vi "Facade.vi"(0 "Data In":T4, 2 "Display State In":T2, 3 "Container State":T3) -> (6 "Data Out":T4, 7 "Display State Out":T2, 8 "Action":T1)   [LabVIEW 2016, in "MGI Path Selector.xctl"]
doc: "Facade VI for the Path Selector XControl. This XControl allows the user to select a path using a combobox. The behavior of the XControl depends upon the LVObject used for its implementation.\n\nAuthored by Shawn Walpole\nsupport@mooregoodideas.com\nwww.mooregoodideas.com\n\nCopyright (c) 2013, Moore Good Ideas, Inc.\n\nAll rights reserved.\n\nRedistribution and use in source and binary forms, with or without modification, are permitted provided that the following conditions are met:\n\n * Redistributions of source code must retain the above copyright notice, this list of conditions and the following disclaimer.\n * Redistributions in binary form must reproduce the above copyright notice, this list of conditions and the following disclaimer in the documentation and/or other materials provided with the distribution.\n * Neither the name of Moore Good Ideas, Inc. nor the names of its contributors may be used to endorse or promote products derived from this software without specific prior written permission.\n\nTHIS SOFTWARE IS PROVIDED BY THE COPYRIGHT HOLDERS AND CONTRIBUTORS \"AS IS\" AND ANY EXPRESS OR IMPLIED WARRANTIES, INCLUDING, BUT NOT LIMITED TO, THE IMPLIED WARRANTIES OF MERCHANTABILITY AND FITNESS FOR A PARTICULAR PURPOSE ARE DISCLAIMED. IN NO EVENT SHALL THE COPYRIGHT OWNER OR CONTRIBUTORS BE LIABLE FOR ANY DIRECT, INDIRECT, INCIDENTAL, SPECIAL, EXEMPLARY, OR CONSEQUENTIAL DAMAGES (INCLUDING, BUT NOT LIMITED TO, PROCUREMENT OF SUBSTITUTE GOODS OR SERVICES; LOSS OF USE, DATA, OR PROFITS; OR BUSINESS INTERRUPTION) HOWEVER CAUSED AND ON ANY THEORY OF LIABILITY, WHETHER IN CONTRACT, STRICT LIABILITY, OR TORT (INCLUDING NEGLIGENCE OR OTHERWISE) ARISING IN ANY WAY OUT OF THE USE OF THIS SOFTWARE, EVEN IF ADVISED OF THE POSSIBILITY OF SUCH DAMAGE."
uses:
  <userlib>/_MGI/User Interface/Path Selector XControl/MGI Path Selector.xctl
  <vilib>/_xctls/Action.ctl
  <vilib>/_xctls/XControlSupport.lvlib
  <userlib>/_MGI/User Interface/Path Selector XControl/Class Hierarchy/MGI Path Selector.lvclass
  <vilib>/event_ctls.llb/lveventtype.ctl
  <userlib>/_MGI/User Interface/Path Selector XControl/Event Cluster.ctl
  <vilib>/Utility/miscctls.llb/LVPoint32TypeDef.ctl
  <vilib>/_xctls/Container State.ctl
  <userlib>/_MGI/User Interface/Path Selector XControl/Data.ctl
  <userlib>/_MGI/User Interface/Path Selector XControl/State.ctl
panel:
  in  "Silver Combo":string(combo)
  in  "Classic Combo":string(combo)
  in  "3D Combo":string(combo)
  in  "Combo Box":string(combo)
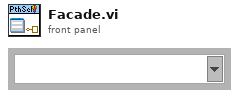
[diagram p1: front panel]
types:
  T1 = typedef "XControlSupport.lvlib/Action.ctl" = cluster{"Data Changed?":bool, "State Changed?":bool, "Action Name":string}
  T2 = typedef "MGI Path Selector.xctl/State.ctl" = cluster{"Class":refnum<class "MGI Path Selector.lvclass">, "Persist":string}
  T3 = typedef "XControlSupport.lvlib/Container State.ctl" = cluster{"Indicator?":bool, "Run Mode?":bool, " Refnum":refnum<vi>}
  T4 = typedef "MGI Path Selector.xctl/Data.ctl" = path
  T5 = typedef "MGI Path Selector.xctl/Event Cluster.ctl" = cluster{"Type":T6, "Combo Box Ref":refnum<vi>, "MenuRef":refnum<k9>, "Coords":T7, "Item Path":string, "Item Tag":string}
  T6 = typedef "lveventtype.ctl" = enum32{"Null", "Timeout", "Annotation Menu Selection", "Annotation Menu Selection?", "App Instance Close", "App Instance Close?", "Autoscale Range Change", "Bookmark Info Change", "Cell Edit", "Cell Edit?", "Cursor Grab", "Cursor Grab?", "Cursor Menu Selection", "Cursor Menu Selection?", "Cursor Move", "Cursor Release", "Data Change", "Direction Change", "Display State Change", "Drag Ended", "Drag Enter", "Drag Leave", "Drag Over", "Drag Source Update", "Drag Starting", "Drag Starting?", "Drop", "Exec State Change", "Key Down", "Key Down?", "Key Repeat", "Key Repeat?", "Key Up", "Listbox Double Click", "Menu Activation?", "Menu Selection (App)", "Menu Selection? (App)", "Menu Selection (User)", "Mouse Down", "Mouse Down?", "Mouse Enter", "Mouse Leave", "Mouse Move", "Mouse Up", "Mouse Wheel", "NI Security User Change (App)", "Pane Size", "Panel Close", "Panel Close?", "Panel Resize", "Plot Attribute Change", "Scale Range Change", "Shortcut Menu Activation?", "Shortcut Menu Selection (App)", "Shortcut Menu Selection? (App)", "Shortcut Menu Selection (User)", "Tree Double Click", "Tree Drag", "Tree Drag?", "Tree Drop", "Tree Drop?", "Tree Item Close", "Tree Item Close?", "Tree Item Open", "Tree Item Open?", "User Event", "Value Change"}
  T7 = typedef "LVPoint32TypeDef.ctl" = cluster{"Horizontal":i32, "Vertical":i32}
  T8 = typedef "MGI Path Selector.xctl/Control Style Enum.ctl" = enum16{"System", "Modern", "Classic", "Silver"}
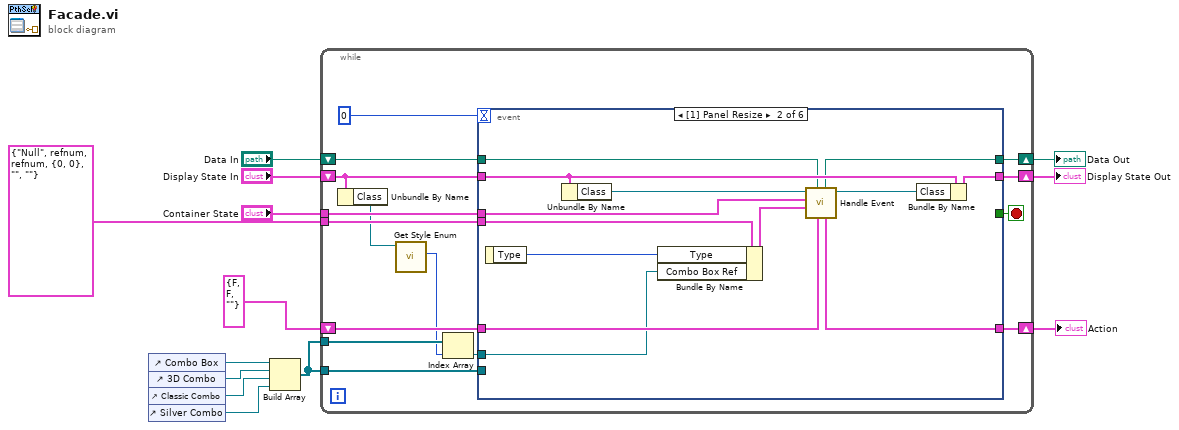
[diagram p0: block diagram]
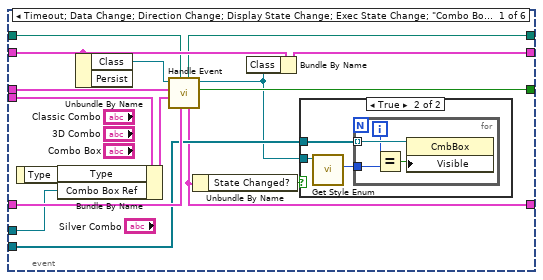
[diagram p2: hidden frame]
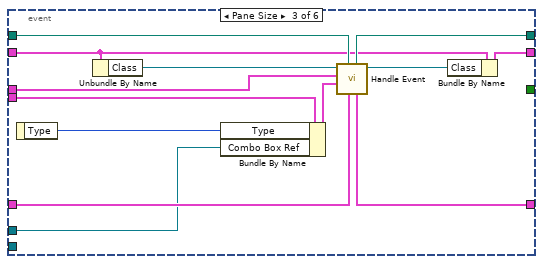
[diagram p4: hidden frame]
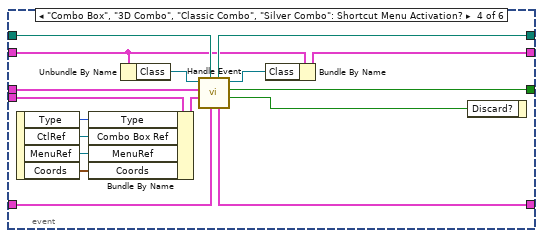
[diagram p5: hidden frame]
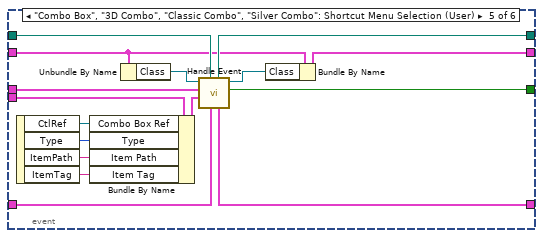
[diagram p6: hidden frame]
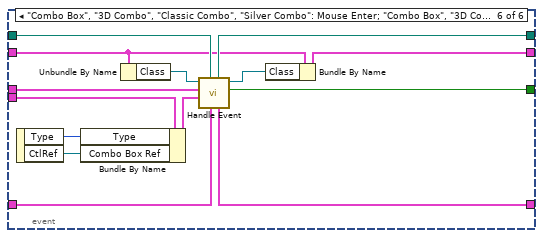
[diagram p7: hidden frame]
diagram:
  n1 = control-ref of="Combo Box"() -> (w5:refnum<vi>)
  n2 = control-ref of="3D Combo"() -> (w4:refnum<vi>)
  n3 = control-ref of="Classic Combo"() -> (w3:refnum<vi>)
  n4 = control-ref of="Silver Combo"() -> (w1:refnum<vi>)
  n5 = Build Array(w5, w4, w3, w1) -> (w2:refnum<vi>[])
  n6 = while {
    shift-right: [w28] -> w10
    shift-left: "Display State In" -> [w18]
    tunnel: "Container State" -> [w25]
    shift-right: [w23] -> w13
    shift-left: "Data In" -> [w24]
    shift-right: [w21] -> w8
    shift-left: T1 {"Data Changed?"=FALSE, "State Changed?"=FALSE, "Action Name"=""} ("Action") -> [w22]
    tunnel: T5 {"Type"=enum."Null", "Combo Box Ref"=refnum, "MenuRef"=refnum, "Coords"={"Horizontal"=0, "Vertical"=0}, "Item Path"="", "Item Tag"=""} ("Event Cluster") -> [w20]
    tunnel: w2 -> [w19]
    tunnel: w2 -> [w16]
    stop <- w27 stop-if-true
    n7 = Unbundle By Name(w18) -> ("Class"=w15:refnum<class "MGI Path Selector.lvclass">)
    n8 = call-dynamic "Get Style Enum.vi"("Path Selector in"=w15) -> ("Control Style"=w14:T8)  [unwired: 10 in]
    n9 = Index Array(array=w19, index=w14) -> (element=w17:refnum<vi>)
    n10 = event shown="[1] Panel Resize" {
      selector: _ -> [_ _ _ _ _ _]
      dyn-events: _ -> [_ _ _ _ _ _]
      timeout: 0 -> [_ _ _ _ _ _]
      tunnel: w18 -> [w43 w64 w74 w86 w103 w117]
      tunnel: [w42 w63 w73 w84 w101 w115] -> w28
      tunnel: [w38 _ _ w90 w106 w120] -> w27
      tunnel: w25 -> [w39 w60 w68 w94 w110 w124]
      tunnel: w24 -> [w33 w55 w76 w93 w109 w123]
      tunnel: [w32 w56 w75 w88 w105 w119] -> w23
      tunnel: [w30 w52 w70 w91 w107 w121] -> w21
      tunnel: w22 -> [w44 w62 w71 w92 w108 w122]
      tunnel: w20 -> [w41 w61 w69 w83 w100 w114]
      tunnel: w17 -> [w35 w57 w65 _ _ _]
      tunnel: w16 -> [w36 _ _ _ _ _]
      event Timeout; Data Change; Direction Change; Display State Change; Exec State Change; "Combo Box", "3D Combo", "Classic Combo", "Silver Combo": Value Change {
        n11 = event-data() -> ("Type"=w37:T6)  [unwired: 1 in]
        n12 = Bundle By Name(cluster=w41, "Type"=w37, "Combo Box Ref"=w35) -> (w40:T5)
        n13 = Unbundle By Name(w43) -> ("Class"=w31:refnum<class "MGI Path Selector.lvclass">)  [unwired: 1 out]
        n14 = call-dynamic "Handle Event.vi"("Action in"=w44, "Data in"=w33, "Event Cluster"=w40, "Container State"=w39, "Path Selector in"=w31) -> ("Facade complete?"=w38:bool, "Path Selector out"=w34:refnum<class "MGI Path Selector.lvclass">, "Action out"=w30:T1, "Data out"=w32:path)  [unwired: 2 in, 1 out]
        n15 = Unbundle By Name(w30) -> ("State Changed?"=w29:bool)
        n16 = Bundle By Name(cluster=w43, "Class"=w34) -> (w42:T2)
        n17 = case shown="True" w29 {
          tunnel: w34 -> [_ w46]
          tunnel: w36 -> [_ w47]
          frame False {
          }
          frame True {
            n18 = call-dynamic "Get Style Enum.vi"("Path Selector in"=w46) -> ("Control Style"=w45:T8)  [unwired: 10 in]
            n19 = for {
              tunnel: w47 -> [w51] mode=indexing
              tunnel: w45 -> [w48]
              i -> [w50]
              n20 = Equal?(x=w50, y=w48) -> (x = y?=w49:bool)
              n21 = property class="CmbBox"(reference=w51, "Visible"=w49) -> ()  [unwired: 1 in, 2 out]
            }
          }
        }
      }
      event Panel Resize {
        n22 = event-data() -> ("Type"=w58:T6)  [unwired: 1 in]
        n23 = Unbundle By Name(w64) -> ("Class"=w53:refnum<class "MGI Path Selector.lvclass">)
        n24 = Bundle By Name(cluster=w61, "Type"=w58, "Combo Box Ref"=w57) -> (w59:T5)
        n25 = call-dynamic "Handle Event.vi"("Action in"=w62, "Data in"=w55, "Event Cluster"=w59, "Container State"=w60, "Path Selector in"=w53) -> ("Path Selector out"=w54:refnum<class "MGI Path Selector.lvclass">, "Action out"=w52:T1, "Data out"=w56:path)  [unwired: 2 in, 2 out]
        n26 = Bundle By Name(cluster=w64, "Class"=w54) -> (w63:T2)
      }
      event Pane Size {
        n27 = event-data() -> ("Type"=w66:T6)  [unwired: 1 in]
        n28 = Unbundle By Name(w74) -> ("Class"=w77:refnum<class "MGI Path Selector.lvclass">)
        n29 = Bundle By Name(cluster=w69, "Type"=w66, "Combo Box Ref"=w65) -> (w67:T5)
        n30 = call-dynamic "Handle Event.vi"("Action in"=w71, "Data in"=w76, "Event Cluster"=w67, "Container State"=w68, "Path Selector in"=w77) -> ("Path Selector out"=w72:refnum<class "MGI Path Selector.lvclass">, "Action out"=w70:T1, "Data out"=w75:path)  [unwired: 2 in, 2 out]
        n31 = Bundle By Name(cluster=w74, "Class"=w72) -> (w73:T2)
      }
      event "Combo Box", "3D Combo", "Classic Combo", "Silver Combo": Shortcut Menu Activation? {
        n32 = event-data() -> ("Type"=w82:T6, "CtlRef"=w80:refnum<vi>, "MenuRef"=w79:refnum<k9>, "Coords"=w78:T7)  [unwired: 1 in]
        n33 = Bundle By Name(cluster=w83, "Type"=w82, "Combo Box Ref"=w80, "MenuRef"=w79, "Coords"=w78) -> (w81:T5)
        n34 = Unbundle By Name(w86) -> ("Class"=w87:refnum<class "MGI Path Selector.lvclass">)
        n35 = call-dynamic "Handle Event.vi"("Action in"=w92, "Data in"=w93, "Event Cluster"=w81, "Container State"=w94, "Path Selector in"=w87) -> ("Discard?"=w89:bool, "Facade complete?"=w90:bool, "Path Selector out"=w85:refnum<class "MGI Path Selector.lvclass">, "Action out"=w91:T1, "Data out"=w88:path)  [unwired: 2 in]
        n36 = Bundle By Name(cluster=w86, "Class"=w85) -> (w84:T2)
        n37 = event-data("Discard?"=w89) -> ()  [unwired: 1 in, 1 out]
      }
      event "Combo Box", "3D Combo", "Classic Combo", "Silver Combo": Shortcut Menu Selection (User) {
        n38 = event-data() -> ("CtlRef"=w98:refnum<vi>, "Type"=w99:T6, "ItemPath"=w97:string, "ItemTag"=w96:string)  [unwired: 1 in]
        n39 = Bundle By Name(cluster=w100, "Combo Box Ref"=w98, "Type"=w99, "Item Path"=w97, "Item Tag"=w96) -> (w95:T5)
        n40 = Unbundle By Name(w103) -> ("Class"=w104:refnum<class "MGI Path Selector.lvclass">)
        n41 = call-dynamic "Handle Event.vi"("Action in"=w108, "Data in"=w109, "Event Cluster"=w95, "Container State"=w110, "Path Selector in"=w104) -> ("Facade complete?"=w106:bool, "Path Selector out"=w102:refnum<class "MGI Path Selector.lvclass">, "Action out"=w107:T1, "Data out"=w105:path)  [unwired: 2 in, 1 out]
        n42 = Bundle By Name(cluster=w103, "Class"=w102) -> (w101:T2)
      }
      event "Combo Box", "3D Combo", "Classic Combo", "Silver Combo": Mouse Enter; "Combo Box", "3D Combo", "Classic Combo", "Silver Combo": Mouse Leave {
        n43 = event-data() -> ("Type"=w113:T6, "CtlRef"=w112:refnum<vi>)  [unwired: 1 in]
        n44 = Bundle By Name(cluster=w114, "Type"=w113, "Combo Box Ref"=w112) -> (w111:T5)
        n45 = Unbundle By Name(w117) -> ("Class"=w118:refnum<class "MGI Path Selector.lvclass">)
        n46 = call-dynamic "Handle Event.vi"("Action in"=w122, "Data in"=w123, "Event Cluster"=w111, "Container State"=w124, "Path Selector in"=w118) -> ("Facade complete?"=w120:bool, "Path Selector out"=w116:refnum<class "MGI Path Selector.lvclass">, "Action out"=w121:T1, "Data out"=w119:path)  [unwired: 2 in, 1 out]
        n47 = Bundle By Name(cluster=w117, "Class"=w116) -> (w115:T2)
      }
    }
  }
  "Display State Out" <- w10
  "Data Out" <- w13
  "Action" <- w8
